vi "start.vi"(8 "error in (no error)":errorcluster, 11 "CameraControlViewer in":refnum<class "CameraControlViewer.lvclass">) -> (0 "error out":errorcluster, 3 "CameraControlViewer out":refnum<class "CameraControlViewer.lvclass">)   [LabVIEW 2011, in "Views.lvlib" / "Camera.lvlib" / "CameraControlViewer.lvclass"]
uses:
  CameraControlViewer.lvclass
  CameraControlViewer.lvclass/CameraControlViewer.ctl
  Hal/HWController/HWControllerEvents/HWControllerEvents.lvclass
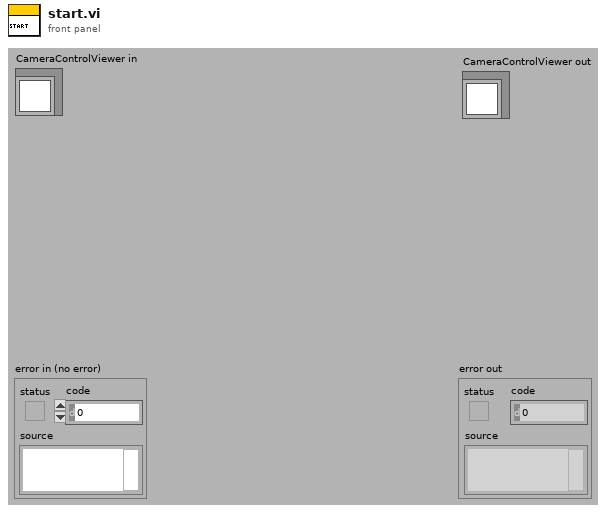
[diagram p1: front panel]
types:
  T1 = enum16{"start", "stop", "statusInquiry", "configure", "resetError", "resourcesInquiry", "reserveResources", "initialise", "resetAllChannels", "staticUpdate", "close", "HWStatus", "error", "resourcesAvailable", "resourcesReserved", "compilerError", "compiledScript", "compilingScript", "runScript", "configureCompiledScript", "restartCompiler", "staticRfChannelUpdate", "cameraUpdate"}
  T2 = cluster{"incomingEventTypes":cluster{"start":cluster{"Boolean":bool}, "stop":cluster{"Boolean":bool}, "statusInquiry":cluster{"Boolean":bool}, "configure":cluster{"DPScriptPath":path, "TimeStamp":string, "HWLoop?":bool}, "resetError":cluster{"Boolean":bool}, "resourcesInquiry":cluster{"Boolean":bool}, "reserveResources":cluster{"HWList":string[]}, "initialise":cluster{"HWList":string[]}, "close":cluster{"Boolean":bool}, "resetAllChannels":cluster{"Boolean":bool}, "staticChannelUpdate":cluster{"channel_address":string, "calibratedValue":dbl}, "runScript":cluster{"DPScriptPath":path, "TimeStamp":string, "HWLoop?":bool}, "compilingScript":cluster{"Path":path}, "compiledScript":cluster{"Path":path, "timeCompileAt":string}, "compilerError":cluster{"Path":path}, "configureCompiledScript":cluster{"DPScriptPath":path, "TimeStamp":string, "HWLoop?":bool, "CompiledScript":cluster{"ScriptListCompiler.lvclass":refnum<class "ScriptListCompiler.lvclass">, "aoChannels":refnum<class "AnalogOutput.lvclass">[], "doChannels":refnum<class "DigitalOutput.lvclass">[], "rfChannels":refnum<class "DDSOutput.lvclass">[]}}, "restartCompiler":cluster{"restart":bool}, "staticRfChannelUpdate":cluster{"channel_address":string, "Output":cluster{"Frequency(MHz)":dbl, "Amplitude":dbl, "Phase":dbl, "OutputForm":enum16{"Sine", "Square", "Triangle", "Arbitrary"}}}, "cameraUpdate":cluster{"Camera":string, "Type":string, "settings":path}}, "outgoingEventTypes":cluster{"HWStatus":cluster{"status":enum16{"Ready", "Compiling", "Configured", "Running", "Stopping", "Unresolved Error"}}, "error":cluster{"error out":errorcluster}, "resourcesAvailable":cluster{"availableHWList":string[], "reservedHWList":string[]}, "resourcesReserved":cluster{"reservedHWList":string[]}}}
  T3 = cluster{"Camera":string, "Type":string, "settings":path}
  T4 = cluster{"eventId":enum16{"start", "stop", "statusInquiry", "configure", "resetError", "resourcesInquiry", "reserveResources", "initialise", "resetAllChannels", "staticUpdate", "close", "HWStatus", "error", "resourcesAvailable", "resourcesReserved", "compilerError", "compiledScript", "compilingScript", "runScript", "configureCompiledScript", "restartCompiler", "staticRfChannelUpdate", "cameraUpdate"}, "cameraUpdate":cluster{"Camera":string, "Type":string, "settings":path}}
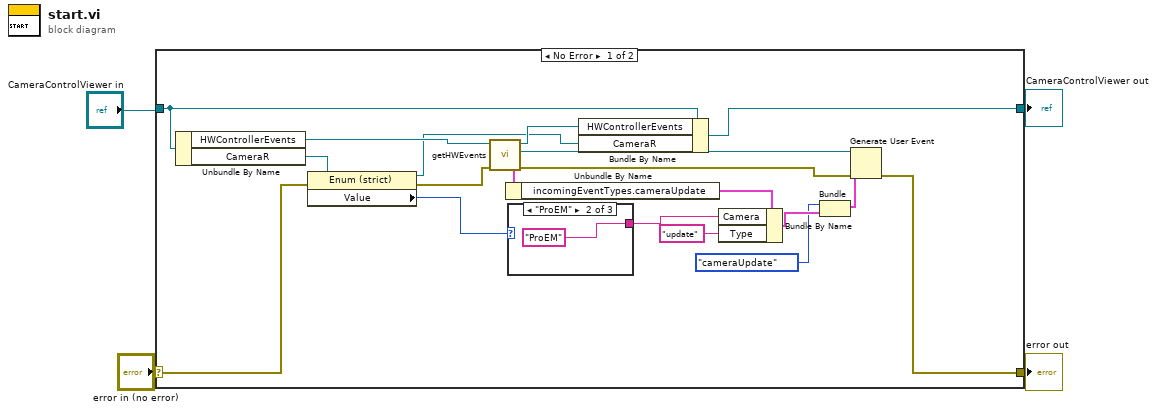
[diagram p0: block diagram]
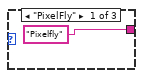
[diagram p2: hidden frame]
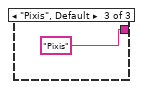
[diagram p3: hidden frame]
diagram:
  n1 = case shown="No Error" "error in (no error)" {
    selector: "error in (no error)" -> [w7 w28]
    tunnel: [w13 w28] -> w3
    tunnel: [w10 w27] -> w1
    tunnel: "CameraControlViewer in" -> [w11 w27]
    frame No Error {
      n2 = Unbundle By Name(w11) -> ("HWControllerEvents"=w23:refnum<class "HWControllerEvents.lvclass">, "CameraR"=w9:refnum<vi>)
      n3 = property class="Enum (strict)"(reference=w9, error in=w7) -> (reference out=w5:refnum<vi>, error out=w6:errorcluster, "Value"=w8:enum16{"Pixis", "ProEM", "PixelFly"})
      n4 = call-dynamic "getHWEvents.vi"("error in (no error)"=w6, "HWControllerEvents in"=w23) -> ("error out"=w17:errorcluster, "eventDataTypes"=w22:T2, "HWCEvent"=w18:refnum<user-event>, "HWControllerEvents out"=w12:refnum<class "HWControllerEvents.lvclass">)  [unwired: 6 in]
      n5 = Unbundle By Name(w22) -> ("incomingEventTypes.cameraUpdate"=w21:T3)
      n6 = case shown="\"ProEM\"" w8 {
        tunnel: ["Pixelfly" "ProEM" "Pixis"] -> w19
        frame "PixelFly" {
        }
        frame "ProEM" {
        }
        frame "Pixis", Default {
        }
      }
      n7 = Bundle By Name(cluster=w11, "HWControllerEvents"=w12, "CameraR"=w5) -> (w10:refnum<class "CameraControlViewer.lvclass">)
      n8 = Bundle By Name(cluster=w21, "Camera"=w19, "Type"="update") -> (w16:T3)
      n9 = Bundle("eventId"=T1."cameraUpdate", "cameraUpdate"=w16) -> (w14:T4)  [unwired: 1 in]
      n10 = Generate User Event(user event=w18, event data cluster=w14, error in=w17) -> (error out=w13:errorcluster)  [unwired: 1 out]
    }
    frame Error {
    }
  }
  "error out" <- w3
  "CameraControlViewer out" <- w1
